vi "rpc_tsmaster_cmd_write_signal.vi"(6 "AValue":dbl, 7 "ABusType":u32(ring) items=["APP_CAN", "APP_LIN", "APP_FlexRay", "APP_Ethernet"], 8 "error in (no error)":errorcluster caption="错误输入（无错误）", 9 "AHandle":u32, 10 "AAddr":string, 11 "路径输入":path) -> (0 "error out":errorcluster caption="错误输出", 2 "function return":i32, 3 "路径输出":path)   [LabVIEW 2014]
doc: "TSAPI(s32)rpc_tsmaster_cmd_write_signal(const size_t AHandle,const TLIBApplicationChannelType ABusType,const char* AAddr,const double AValue);"
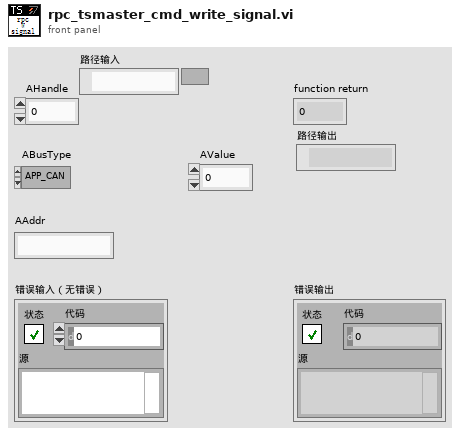
[diagram p1: front panel]
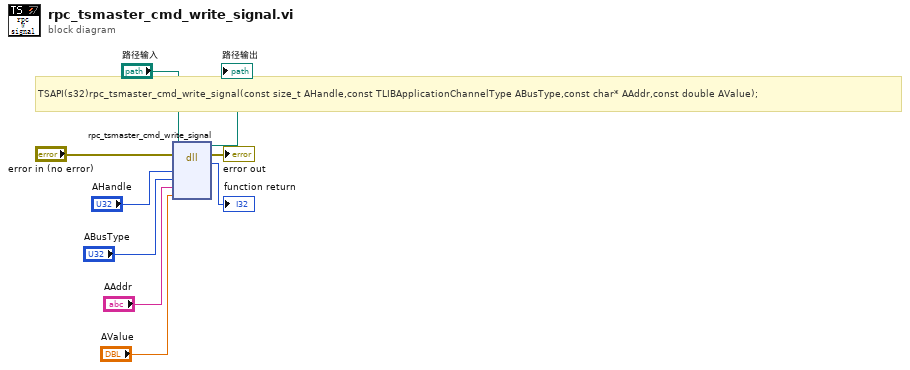
[diagram p0: block diagram]
diagram:
  # "TSAPI(s32)rpc_tsmaster_cmd_write_signal(const size_t AHandle,const TLIBApplicationChannelType ABusType,const char* AAddr,const double AValue);"
  n1 = dll-call lib="D:/Work/LabVIEW Code/TSMaster Labview SDK/LabVIEW/LabVIEW-TSMasterAPI_CLN/TSMasterAPI_LabVIEW-2024-10-08 14-20-13/Not_organized_vi/TSMaster.*" fn="rpc_tsmaster_cmd_write_signal"(path in="路径输入", error in="error in (no error)", "AHandle"="AHandle", "ABusType"="ABusType", "AAddr"="AAddr", "AValue"="AValue") -> (path out=→"路径输出":path, error out=→"error out":errorcluster, "返回类型"=→"function return":i32)  [unwired: 5 in]
